vi "Drop Message Static.vi"(11 "Message in":refnum<class "Message.lvclass">) -> ()   [LabVIEW 2022 SP3, in "Artifex.lvlib" / "Message.lvclass"]
uses:
  Message.lvclass
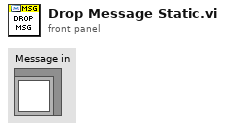
[diagram p1: front panel]
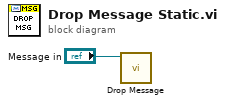
[diagram p0: block diagram]
diagram:
  n1 = call-dynamic "Drop Message.vi"("Message in"="Message in") -> ()  [unwired: 11 in]
